vi "SetCoordinates.vi"(11 "FPGA VI Reference Out":T1) -> ()   [LabVIEW 2009]
uses:
  <vilib>/rvi/interface/nirviReadWriteControl/nirviReadWriteControl.xnode
  FPGA_Control/AODRef.ctl
  FPGA_Control/FPGA Bitfiles/AOD Control.lvproj_PXIe-7965R_AOD Control (FPGA)~D2.lvbitx
  FPGA_Control/AOD Control (FPGA).vi
panel:
  in  "Set":bool
  in  "stop":bool
  out "Setting":T2
  in  "Offset":T2 {"XHP" format="%x"; "XLP" format="%x"; "YHP" format="%x"; "YLP" format="%x"}
  in  "Center Frequencies":T2={"XHP"=858993459, "XLP"=858993459, "YHP"=858993459, "YLP"=858993459} {"XHP" format="%x"; "XLP" format="%x"; "YHP" format="%x"; "YLP" format="%x"}
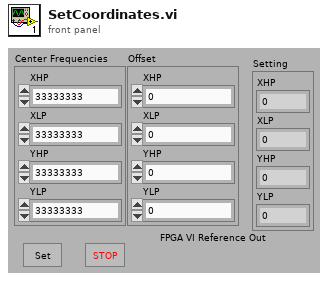
[diagram p1: front panel]
types:
  T1 = typedef "AODRef.ctl" = refnum<k20>
  T2 = cluster{"XHP":i32, "XLP":i32, "YHP":i32, "YLP":i32}
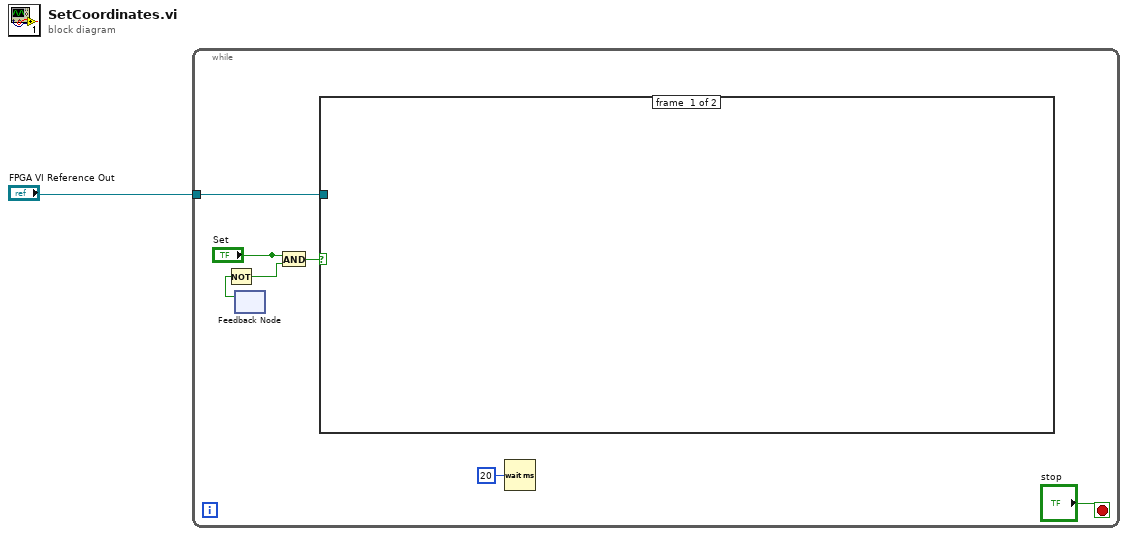
[diagram p0: block diagram]
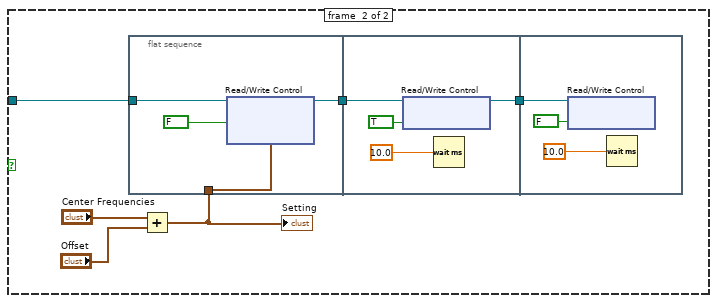
[diagram p2: hidden frame]
diagram:
  n1 = while {
    tunnel: "FPGA VI Reference Out" -> [w7]
    stop <- "stop" stop-if-true
    n2 = feedback #1() -> (w6:bool)  [unwired: 1 in]
    n3 = Not(x=w6) -> (.not. x?=w3:bool)
    n4 = And(x="Set", y=w3) -> (x .and. y?=w5:bool)
    n5 = case shown="True" w5 {
      tunnel: w7 -> [_ w9]
      frame #0 {
      }
      frame #1 {
        n6 = flat-sequence {
          tunnel: w9 -> [w17]
          tunnel: w10 -> [w16]
          tunnel: [w15] -> w14
          tunnel: w14 -> [w37]
          tunnel: [w36] -> w13
          tunnel: w13 -> [w53]
          frame #0 {
            n7 = xnode "Read/Write Control"("FPGA VI Reference In"=w17, "SetCoordinate"=FALSE, "Coordinate"=w16) -> ("FPGA VI Reference Out"=w15:T1)  [unwired: 1 in, 1 out]
          }
          frame #1 {
            n8 = xnode "Read/Write Control"("FPGA VI Reference In"=w37, "SetCoordinate"=TRUE) -> ("FPGA VI Reference Out"=w36:T1)  [unwired: 1 in, 1 out]
            n9 = Wait (ms)(milliseconds to wait=10.0 ("Pause (ms)")) -> ()  [unwired: 1 out]
          }
          frame #2 {
            n10 = xnode "Read/Write Control"("FPGA VI Reference In"=w53, "SetCoordinate"=FALSE) -> ()  [unwired: 1 in, 2 out]
            n11 = Wait (ms)(milliseconds to wait=10.0 ("Pause (ms)")) -> ()  [unwired: 1 out]
          }
        }
        n12 = Add(x="Center Frequencies", y="Offset") -> (x+y=w10:T2)
        "Setting" <- w10
      }
    }
    n13 = Wait (ms)(milliseconds to wait=u32 20) -> ()  [unwired: 1 out]
  }
